vi "Set Target.vi"(3 "Control Mode":T1 items=["PercentOutput"=0, "Position"=1, "Velocity"=2, "Current"=3, "Follower"=5, "MotionProfile"=6, "MotionMagic"=7, "MotionProfileArc"=10, "Disabled"=15], 10 "Input":cluster{"LF":dbl, "LB":dbl, "RF":dbl, "RB":dbl}, 11 "Swerve motors":cluster{"LF":T3, "LB":T3, "RF":T3, "RB":T3}) -> ()   [LabVIEW 2020]
uses:
  <vilib>/Rock Robotics/WPI/MotorControl/WPI_MotorControlDeviceRef.ctl
  <vilib>/Rock Robotics/WPI/MotorControl/WPI_MotorControlType.ctl
  <vilib>/Rock Robotics/SystemInterfaces/DIO/FPGA_DIOPWMChannel.ctl
  <vilib>/Rock Robotics/WPI/PWM/WPI_PWMDeadband.ctl
  <vilib>/Rock Robotics/SystemInterfaces/DIO/FPGA_DIOChannel.ctl
  <vilib>/Rock Robotics/WPI/ThirdParty/Phoenix-LabVIEW/Motor Controller/Controls/CTRE_Phoenix_MotorControl_ControlMode.ctl
  <vilib>/Rock Robotics/WPI/ThirdParty/Phoenix-LabVIEW/Motor Controller/Get/CTRE_Phoenix_MotorController_GetSelectedSensorData.vi
panel:
  in  "PID":bool
  out "RB":T2(graph)
  out "LB":T2(graph)
  out "RF":T2(graph)
  out "LF":T2(graph)
  in  "F":dbl
  in  "D":dbl
  in  "I":dbl
  in  "P":dbl
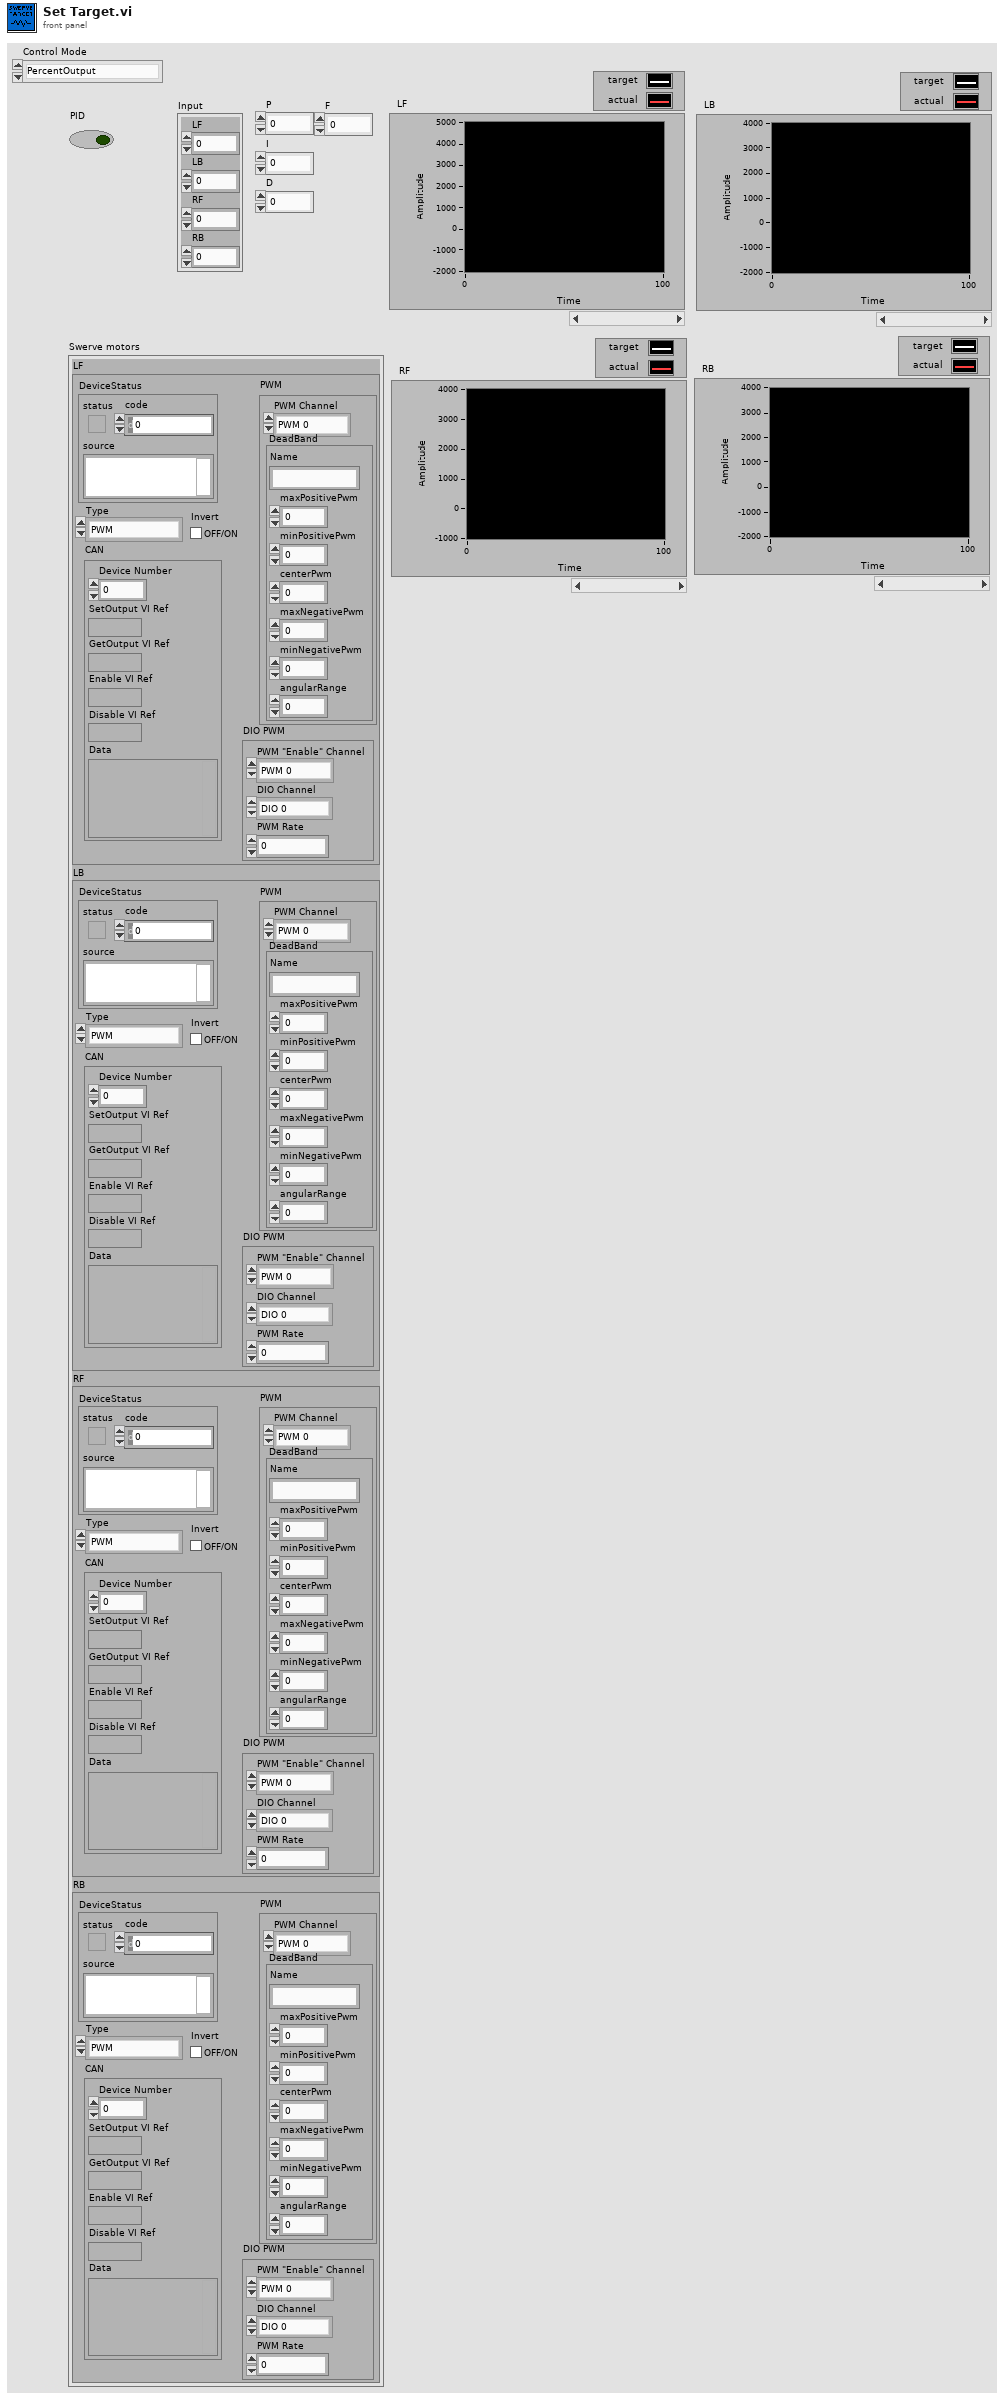
[diagram p1: front panel]
types:
  T1 = typedef "CTRE_Phoenix_MotorControl_ControlMode.ctl" = u16
  T2 = cluster{"Velocity (ticks/ms)":dbl, "Velocity (Raw Sensor Units per 100 ms)":i32}
  T3 = typedef "WPI_MotorControlDeviceRef.ctl" = cluster{"DeviceStatus":errorcluster, "Type":T4, "PWM":cluster{"PWM Channel":T5, "DeadBand":T6}, "CAN":cluster{"Device Number":u8, "SetOutput VI Ref":variant, "GetOutput VI Ref":variant, "Enable VI Ref":variant, "Disable VI Ref":variant, "Data":variant}, "Invert":bool, "DIO PWM":cluster{"PWM \"Enable\" Channel":T5, "DIOChannel":T7, "PWM Rate":dbl}}
  T4 = typedef "WPI_MotorControlType.ctl" = enum16{"PWM", "CAN", "DIO PWM"}
  T5 = typedef "FPGA_DIOPWMChannel.ctl" = enum8{"PWM 0", "PWM 1", "PWM 2", "PWM 3", "PWM 4", "PWM 5", "PWM 6", "PWM 7", "PWM 8", "PWM 9", "PWM MXP 0", "PWM MXP 1", "PWM MXP 2", "PWM MXP 3", "PWM MXP 4", "PWM MXP 5", "PWM MXP 6", "PWM MXP 7", "PWM MXP 8", "PWM MXP 9", "Invalid"}
  T6 = typedef "WPI_PWMDeadband.ctl" = cluster{"Name":string, "maxPositivePwm":i32, "minPositivePwm":i32, "centerPwm":i32, "maxNegativePwm":i32, "minNegativePwm":i32, "angularRange":u16}
  T7 = typedef "FPGA_DIOChannel.ctl" = enum8{"DIO 0", "DIO 1", "DIO 2", "DIO 3", "DIO 4", "DIO 5", "DIO 6", "DIO 7", "DIO 8", "DIO 9", "DIO MXP 0", "DIO MXP 1", "DIO MXP 2", "DIO MXP 3", "DIO MXP 4", "DIO MXP 5", "DIO MXP 6", "DIO MXP 7", "DIO MXP 8", "DIO MXP 9", "DIO MXP 10", "DIO MXP 11", "DIO MXP 12", "DIO MXP 13", "DIO MXP 14", "DIO MXP 15", "SPI Port CS1", "SPI Port CS2", "SPI Port CS3", "SPI Port MISO", "SPI Port MOSI", "Invalid"}
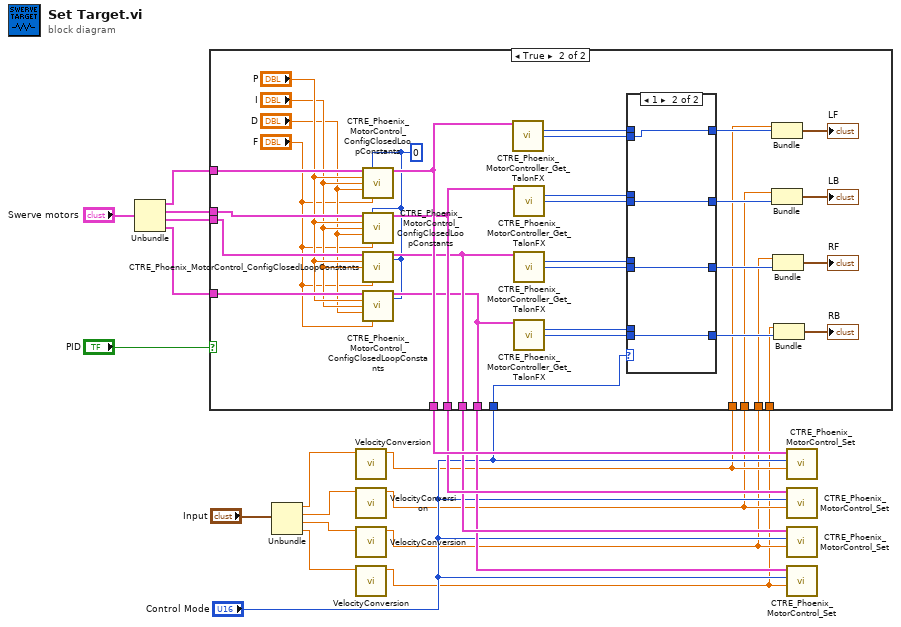
[diagram p0: block diagram]
diagram:
  n1 = Unbundle("Swerve motors") -> ("LF"=w19:T3, "LB"=w18:T3, "RF"=w17:T3, "RB"=w16:T3)
  n2 = Unbundle("Input") -> ("LF"=w14:dbl, "LB"=w13:dbl, "RF"=w12:dbl, "RB"=w11:dbl)
  n3 = call "VelocityConversion.vi"("Velocity (ft/s)"=w14) -> ("Velocity (ticks/ms)"=w5:dbl)  [unwired: 10 in]
  n4 = call "VelocityConversion.vi"("Velocity (ft/s)"=w13) -> ("Velocity (ticks/ms)"=w4:dbl)  [unwired: 10 in]
  n5 = call "VelocityConversion.vi"("Velocity (ft/s)"=w12) -> ("Velocity (ticks/ms)"=w3:dbl)  [unwired: 10 in]
  n6 = call "VelocityConversion.vi"("Velocity (ft/s)"=w11) -> ("Velocity (ticks/ms)"=w2:dbl)  [unwired: 10 in]
  n7 = case shown="True" "PID" {
    tunnel: w19 -> [w24 w58]
    tunnel: w18 -> [w23 w57]
    tunnel: w17 -> [w22 w56]
    tunnel: w16 -> [w21 w55]
    tunnel: [w24 w42] -> w10
    tunnel: [w23 w41] -> w9
    tunnel: [w22 w40] -> w8
    tunnel: [w21 w39] -> w7
    tunnel: "Control Mode" -> [_ w38]
    tunnel: w5 -> [_ w33]
    tunnel: w4 -> [_ w32]
    tunnel: w3 -> [_ w31]
    tunnel: w2 -> [_ w30]
    frame False {
    }
    frame True {
      w25 = 0 ("slotIdx")
      n8 = call <vilib>:"CTRE_Phoenix_MotorControl_ConfigClosedLoopConstants.vi"("PhoenixMotorControlDevRef"=w58, "slotIdx"=w25, "P"="P", "I"="I", "D"="D", "F"="F") -> ("PhoenixMotorControlDevRef"=w42:T3)  [unwired: 8 in, 1 out]
      n9 = call <vilib>:"CTRE_Phoenix_MotorControl_ConfigClosedLoopConstants.vi"("PhoenixMotorControlDevRef"=w57, "slotIdx"=w25, "P"="P", "I"="I", "D"="D", "F"="F") -> ("PhoenixMotorControlDevRef"=w41:T3)  [unwired: 8 in, 1 out]
      n10 = call <vilib>:"CTRE_Phoenix_MotorControl_ConfigClosedLoopConstants.vi"("PhoenixMotorControlDevRef"=w56, "slotIdx"=w25, "P"="P", "I"="I", "F"="F") -> ("PhoenixMotorControlDevRef"=w40:T3)  [unwired: 9 in, 1 out]
      n11 = call <vilib>:"CTRE_Phoenix_MotorControl_ConfigClosedLoopConstants.vi"("PhoenixMotorControlDevRef"=w55, "slotIdx"=w25, "P"="P", "I"="I", "D"="D", "F"="F") -> ("PhoenixMotorControlDevRef"=w39:T3)  [unwired: 8 in, 1 out]
      n12 = call-poly <vilib>:"CTRE_Phoenix_MotorController_Get_TalonFX.vi"("PhoenixMotorControlDevRef"=w42) -> ("Position (Raw Sensor Units)"=w50:i32, "Velocity (Raw Sensor Units per 100 ms)"=w49:i32)  [unwired: 11 in, 2 out]
      n13 = call-poly <vilib>:"CTRE_Phoenix_MotorController_Get_TalonFX.vi"("PhoenixMotorControlDevRef"=w41) -> ("Position (Raw Sensor Units)"=w48:i32, "Velocity (Raw Sensor Units per 100 ms)"=w47:i32)  [unwired: 11 in, 2 out]
      n14 = call-poly <vilib>:"CTRE_Phoenix_MotorController_Get_TalonFX.vi"("PhoenixMotorControlDevRef"=w40) -> ("Position (Raw Sensor Units)"=w46:i32, "Velocity (Raw Sensor Units per 100 ms)"=w45:i32)  [unwired: 11 in, 2 out]
      n15 = call-poly <vilib>:"CTRE_Phoenix_MotorController_Get_TalonFX.vi"("PhoenixMotorControlDevRef"=w39) -> ("Position (Raw Sensor Units)"=w44:i32, "Velocity (Raw Sensor Units per 100 ms)"=w43:i32)  [unwired: 11 in, 2 out]
      n16 = case shown="1" w38 {
        tunnel: w50 -> [w62 _]
        tunnel: w49 -> [_ w66]
        tunnel: w48 -> [_ _]
        tunnel: w47 -> [w61 w65]
        tunnel: w46 -> [_ _]
        tunnel: w45 -> [w60 w64]
        tunnel: w44 -> [_ _]
        tunnel: w43 -> [w59 w63]
        tunnel: [w62 w66] -> w37
        tunnel: [w61 w65] -> w36
        tunnel: [w60 w64] -> w35
        tunnel: [w59 w63] -> w34
        frame 2, Default {
        }
        frame 1 {
        }
      }
      n17 = Bundle("Velocity (ticks/ms)"=w33, "Velocity (Raw Sensor Units per 100 ms)"=w37) -> (→"LF":T2)  [unwired: 1 in]
      n18 = Bundle("Velocity (ticks/ms)"=w32, "Velocity (Raw Sensor Units per 100 ms)"=w36) -> (→"LB":T2)  [unwired: 1 in]
      n19 = Bundle("Velocity (ticks/ms)"=w31, "Velocity (Raw Sensor Units per 100 ms)"=w35) -> (→"RF":T2)  [unwired: 1 in]
      n20 = Bundle("Velocity (ticks/ms)"=w30, "Velocity (Raw Sensor Units per 100 ms)"=w34) -> (→"RB":T2)  [unwired: 1 in]
    }
  }
  n21 = call <vilib>:"CTRE_Phoenix_MotorControl_Set.vi"("Output"=w5, "Control Mode"="Control Mode", "PhoenixMotorControlDevRef"=w10) -> ()  [unwired: 7 in, 2 out]
  n22 = call <vilib>:"CTRE_Phoenix_MotorControl_Set.vi"("Output"=w4, "Control Mode"="Control Mode", "PhoenixMotorControlDevRef"=w9) -> ()  [unwired: 7 in, 2 out]
  n23 = call <vilib>:"CTRE_Phoenix_MotorControl_Set.vi"("Output"=w3, "Control Mode"="Control Mode", "PhoenixMotorControlDevRef"=w8) -> ()  [unwired: 7 in, 2 out]
  n24 = call <vilib>:"CTRE_Phoenix_MotorControl_Set.vi"("Output"=w2, "Control Mode"="Control Mode", "PhoenixMotorControlDevRef"=w7) -> ()  [unwired: 7 in, 2 out]
